vi "Construct log path.vi"(8 "error in":errorcluster, 9 "Log Num":i32, 10 "Append if found?":bool=TRUE, 11 "Log Directory":path) -> (0 "error out":errorcluster, 1 "Log Num out":i32, 2 "exists":bool, 3 "Log file out":path)   [LabVIEW 2018]
uses:
  <userlib>/_OpenG.lib/file/file.llb/File Exists - Scalar__ogtk.vi
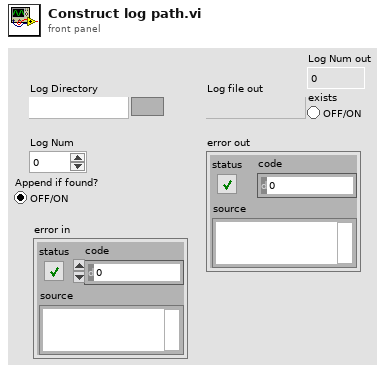
[diagram p1: front panel]
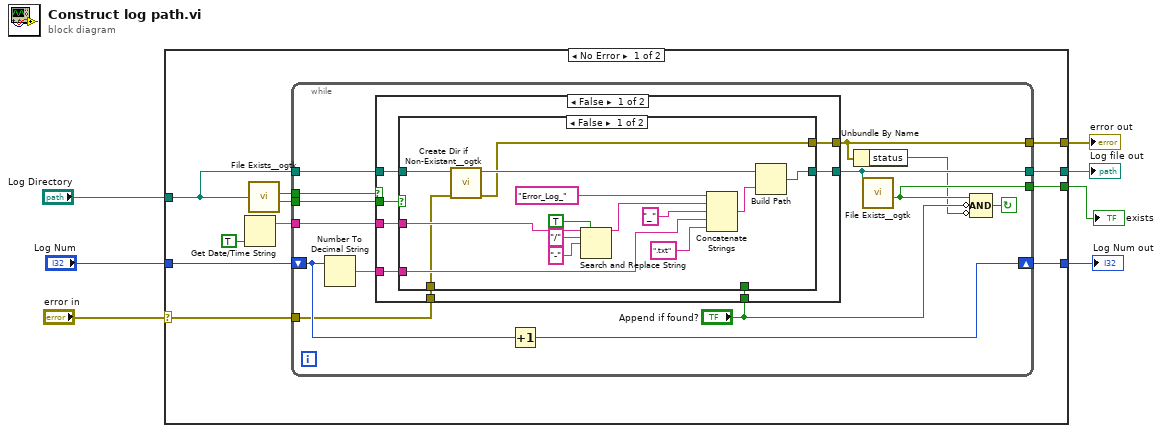
[diagram p0: block diagram]
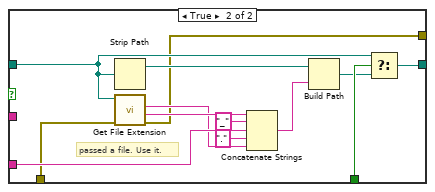
[diagram p2: hidden frame]
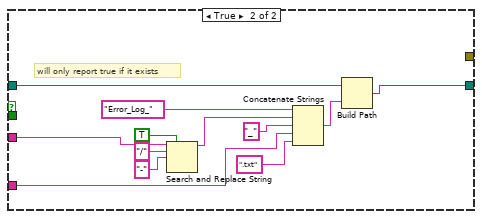
[diagram p3: hidden frame]
diagram:
  n1 = case shown="No Error" "error in" {
    selector: "error in" -> [w8 w82]
    tunnel: [w18 w82] -> w7
    tunnel: [w17 _] -> w6
    tunnel: "Log Directory" -> [w14 _]
    tunnel: "Log Num" -> [w11 w81]
    tunnel: [w10 w81] -> w3
    tunnel: [w9 _] -> w2
    frame No Error {
      n2 = Get Date/Time String(want seconds? (F)=TRUE) -> (date string=w12:string)  [unwired: 2 in, 1 out]
      n3 = call-poly <userlib>:"File Exists__ogtk.vi"("file path"=w14) -> ("is directory"=w15:bool, "exists"=w16:bool)  [unwired: 6 in]
      n4 = while {
        tunnel: [w20] -> w18
        tunnel: w16 -> [w32]
        tunnel: w15 -> [w31]
        tunnel: w12 -> [w29]
        tunnel: w14 -> [w30]
        tunnel: [w28] -> w17
        shift-right: [w25] -> w10
        shift-left: w11 -> [w26]
        tunnel: [w23] -> w9
        tunnel: w8 -> [w21]
        stop <- w24 continue-if-true
        n5 = Number To Decimal String(number=w26) -> (decimal integer string=w27:string)  [unwired: 1 in]
        n6 = case shown="False" w31 {
          tunnel: w30 -> [w40 w73]
          tunnel: w29 -> [w39 w72]
          tunnel: [w38 w71] -> w28
          tunnel: w32 -> [w37 _]
          tunnel: [w35 _] -> w20
          tunnel: w27 -> [w36 w69]
          tunnel: "Append if found?" -> [w34 _]
          tunnel: w21 -> [w33 _]
          frame False {
            n7 = case shown="False" w37 {
              tunnel: w40 -> [w44 w62]
              tunnel: w39 -> [w54 _]
              tunnel: [w47 w63] -> w38
              tunnel: w36 -> [w45 w67]
              tunnel: [w42 w58] -> w35
              tunnel: w34 -> [_ w64]
              tunnel: w33 -> [w41 w56]
              frame False {
                n8 = call <userlib>:"Create Dir if Non-Existant__ogtk.vi"("error in (no error)"=w41, "Directory Path"=w44) -> ("error out"=w42:errorcluster, "dup Directory Path"=w43:path)  [unwired: 7 in, 1 out]
                n9 = Search and Replace String(replace all?=TRUE ("replace all? (F)"), input string=w54, search string="/", replace string="-" ("search string")) -> (result string=w50:string)  [unwired: 4 in, 3 out]
                n10 = Concatenate Strings("Error_Log_" ("string"), w50, "_" ("string"), w45, ".txt" ("string")) -> (w48:string)
                n11 = Build Path(base path=w43, name or relative path=w48) -> (appended path=w47:path)
              }
              frame True {
                # "passed a file. Use it."
                n12 = Strip Path(path=w62) -> (stripped path=w60:path)  [unwired: 1 out]
                n13 = call <vilib>:"Get File Extension.vi"("error in (no error)"=w56, "file"=w62) -> ("error out"=w58:errorcluster, "filename without extension"=w68:string, "lowercase file extension"=w66:string)  [unwired: 5 in, 2 out]
                n14 = Concatenate Strings(w68, "_" ("string"), w67, "." ("string"), w66) -> (w59:string)
                n15 = Build Path(base path=w60, name or relative path=w59) -> (appended path=w61:path)
                n16 = Select(t=w62, s=w64, f=w61) -> (s? t:f=w63:path)
              }
            }
          }
          frame True {
            # "will only report true if it exists"
            n17 = Search and Replace String(replace all?=TRUE ("replace all? (F)"), input string=w72, search string="/", replace string="-" ("search string")) -> (result string=w76:string)  [unwired: 4 in, 3 out]
            n18 = Concatenate Strings("Error_Log_" ("string"), w76, "_" ("string"), w69, ".txt" ("string")) -> (w74:string)
            n19 = Build Path(base path=w73, name or relative path=w74) -> (appended path=w71:path)
          }
        }
        n20 = Increment(x=w26) -> (x+1=w25:i32)
        n21 = Unbundle By Name(w20) -> ("status"=w19:bool)
        n22 = call-poly <userlib>:"File Exists__ogtk.vi"("file path"=w28) -> ("exists"=w23:bool)  [unwired: 6 in, 1 out]
        n23 = Compound Arithmetic op=AND(w23, invert "Append if found?", invert w19) -> (w24:bool)
      }
    }
    frame Error {
    }
  }
  "error out" <- w7
  "Log file out" <- w6
  "Log Num out" <- w3
  "exists" <- w2
